vi "ContinuousCapture.vi"(8 "error in (no error)":errorcluster, 11 "Instruments in":refnum<class "Instruments.lvclass">) -> (0 "error out":errorcluster, 3 "Instruments out":refnum<class "Instruments.lvclass">)   [LabVIEW 2012, in "Instruments.lvclass"]
uses:
  Instruments.lvclass
  Instruments.lvclass/Instruments.ctl
  SpectrumCommands.ctl
  Controls/SpectrometerOphirSelector.ctl
  SpectrumWindowExit.vi
  Controls/Config.ctl
panel:
  in  "DeviceCurrent":enum16{"20mA", "50mA"}(ring)
  out "Vf":dbl format="%0.2f"
  out "Keithley":refnum<visa-resource-name>
  out "DeviceIndicator":bool
  in  "TurnOffDevice":bool
  in  "TurnOnDevice":bool
  out "Ready":bool
  in  "Int Time(ms)":i32
  in  "Enabled":bool
  in  "Exit":bool
  in  "StopCapture":bool
  in  "StartCapture":bool
  in  "Graph":cluster{"Y":dbl[], "Y":dbl[]}[](graph)
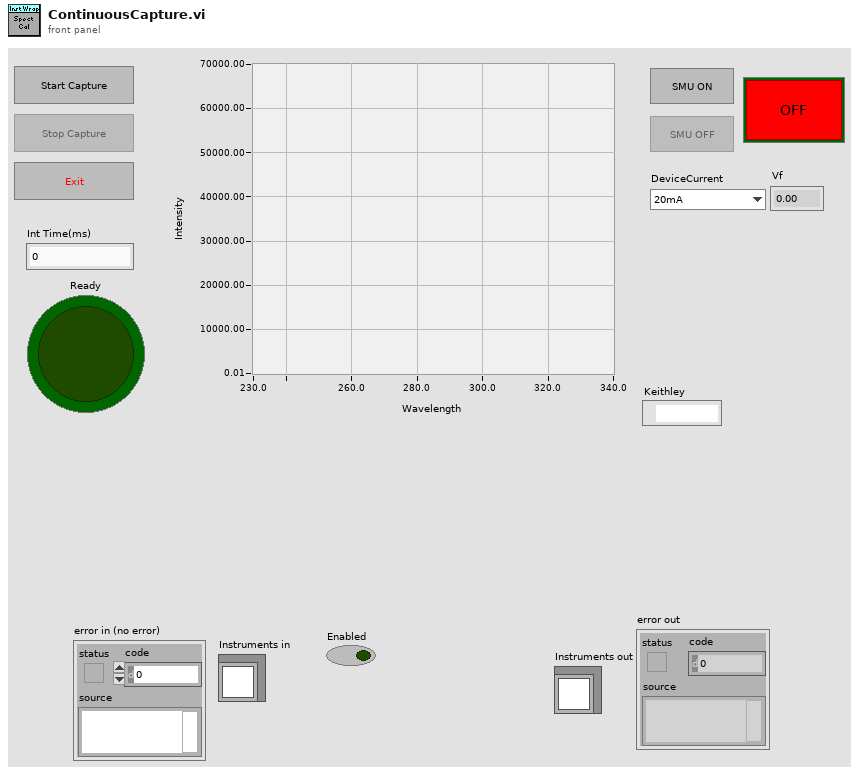
[diagram p1: front panel]
types:
  T1 = enum8{"Enabled", "Disabled", "Disabled and Grayed Out"}
  T2 = cluster{"StopCapture":refnum<vi>, "StartCapture":refnum<vi>, "Exit":refnum<vi>, "Enabled":refnum<vi>, "Ready":refnum<vi>}
  T3 = typedef "Config.ctl" = cluster{"IntTime":i32, "Samples":i32, "PowerMin":dbl, "KneeMin":dbl, "KneeMax":dbl, "Background Wl":dbl, "Settle Delay,ms":u32, "StationId":sgl}
  T4 = typedef "SpectrumCommands.ctl" = enum16{"Init", "StartCapture", "StopCapture", "Calibrate", "TurnDeviceOn", "TurnOffDevice", "Exit"}
  T5 = typedef "SpectrometerOphirSelector.ctl" = enum16{"Get Background", "Measure", "Measure50", "Raw"}
  T6 = cluster{"Wavelength":dbl[], "EL Spectrum":dbl[]}[]
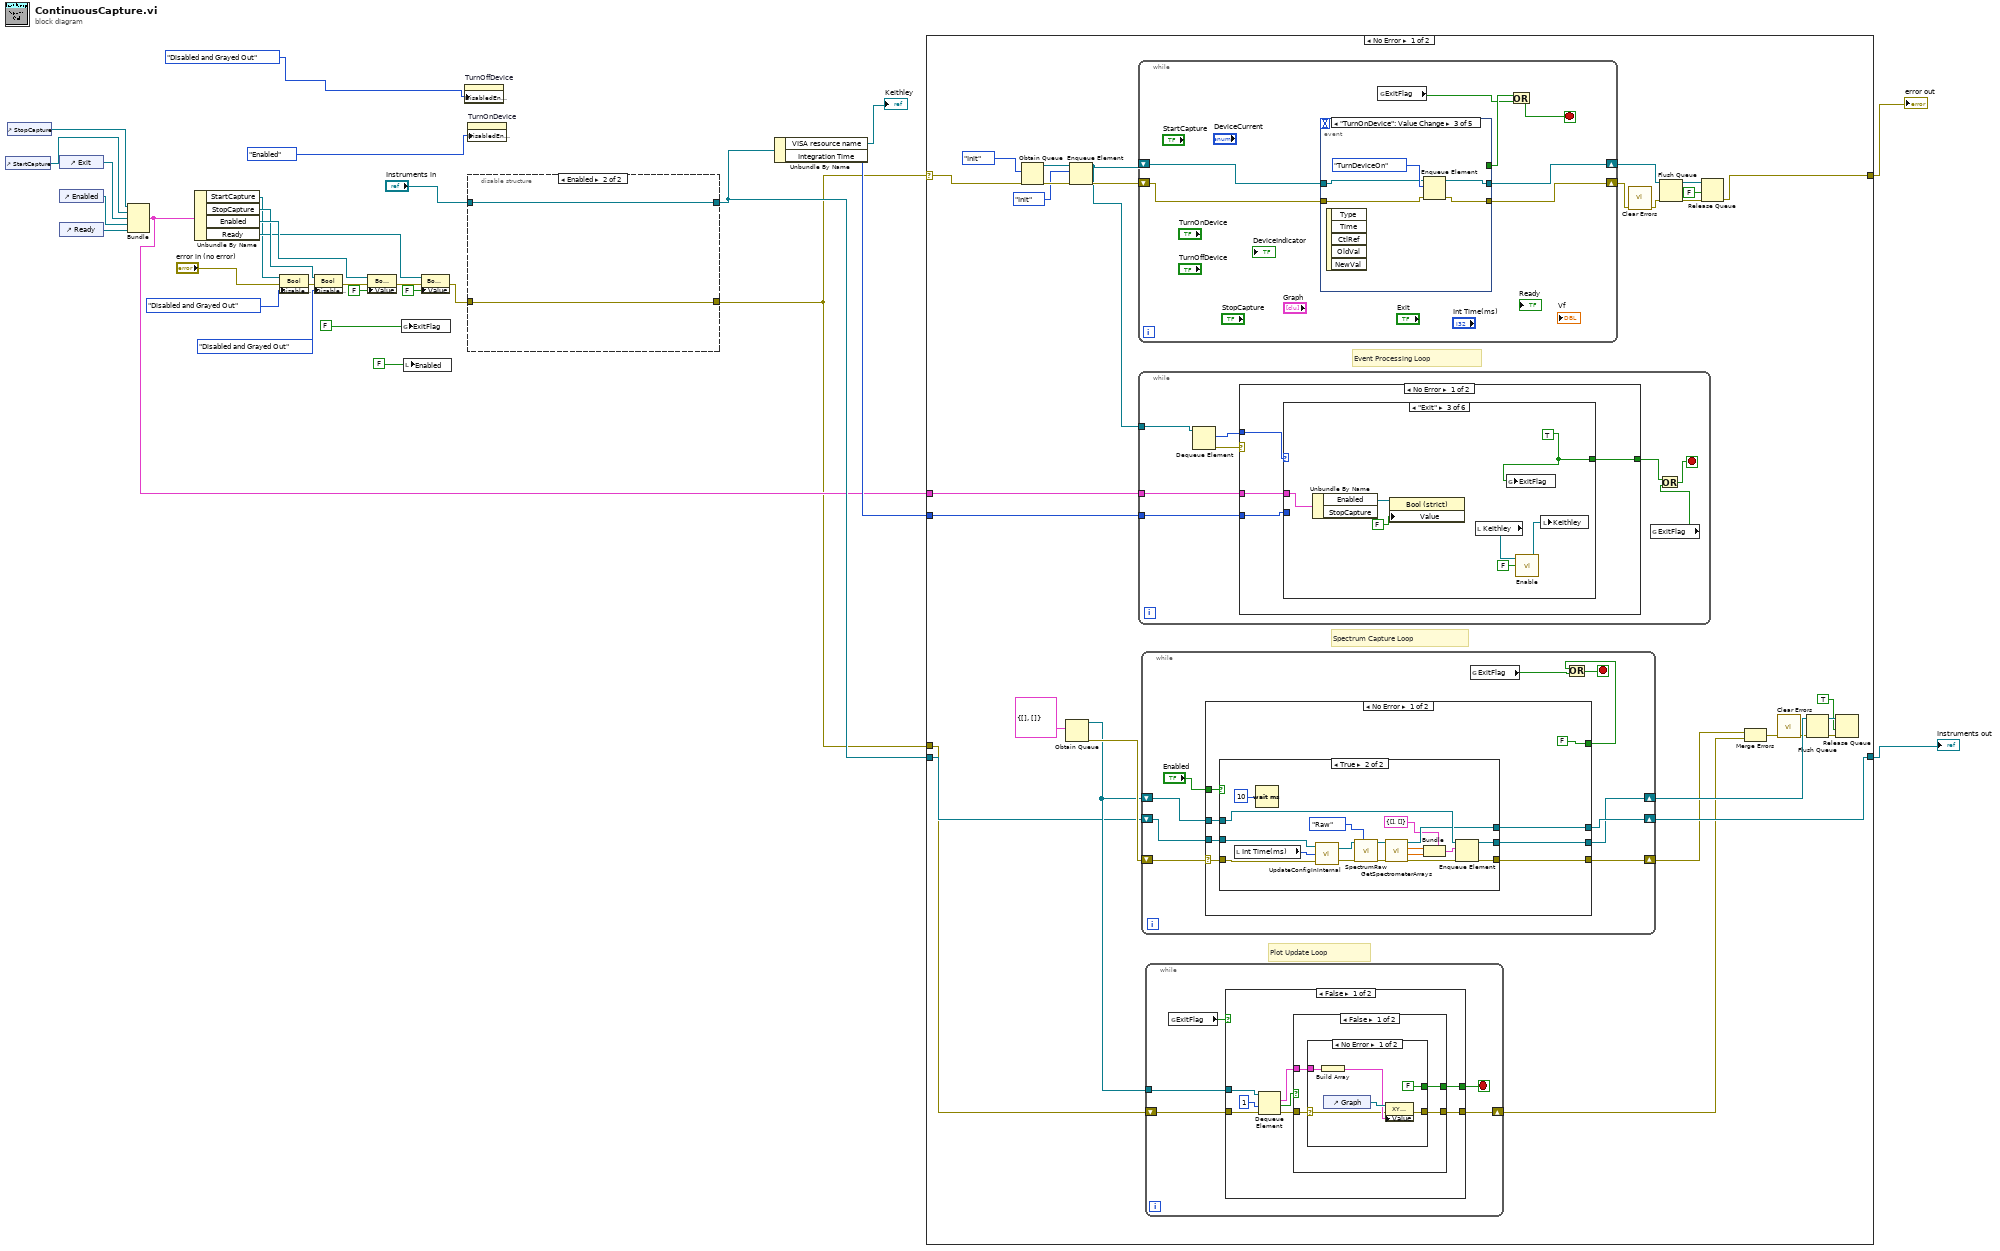
[diagram p0: block diagram]
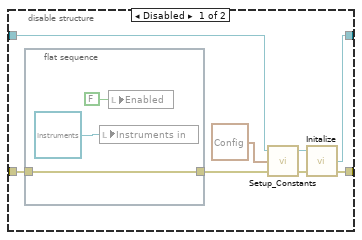
[diagram p2: hidden frame]
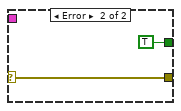
[diagram p3: hidden frame]
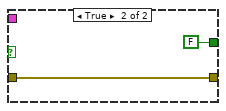
[diagram p4: hidden frame]
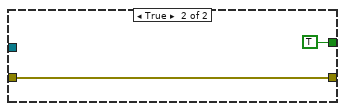
[diagram p5: hidden frame]
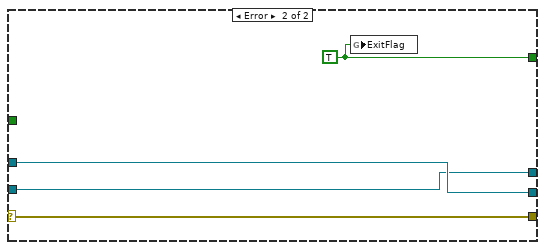
[diagram p7: hidden frame]
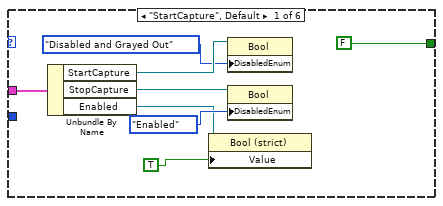
[diagram p8: hidden frame]
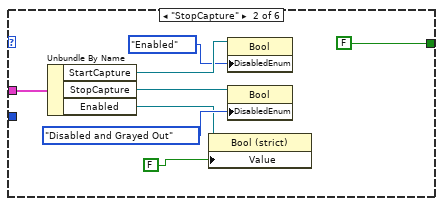
[diagram p9: hidden frame]
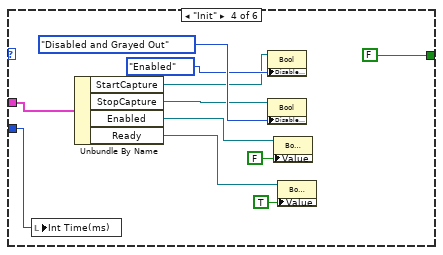
[diagram p10: hidden frame]
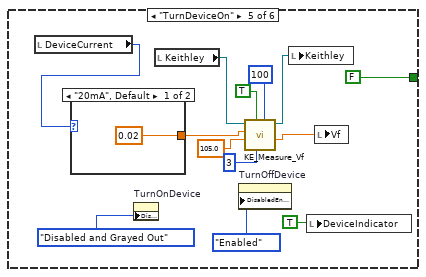
[diagram p11: hidden frame]
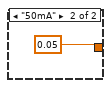
[diagram p12: hidden frame]
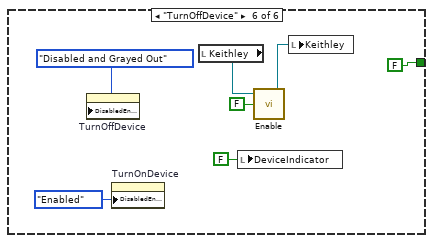
[diagram p13: hidden frame]
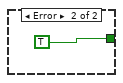
[diagram p14: hidden frame]
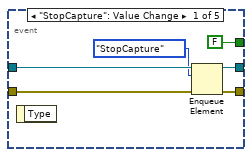
[diagram p15: hidden frame]
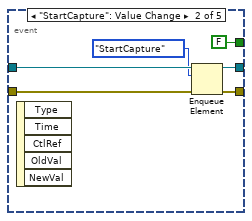
[diagram p16: hidden frame]
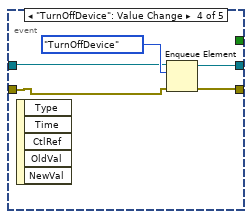
[diagram p17: hidden frame]
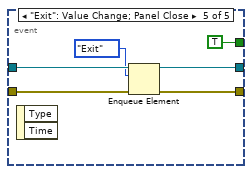
[diagram p18: hidden frame]
diagram:
  n1 = control-ref of="StartCapture"() -> (w27:refnum<vi>)
  n2 = control-ref of="StopCapture"() -> (w28:refnum<vi>)
  n3 = control-ref of="Exit"() -> (w26:refnum<vi>)
  n4 = control-ref of="Enabled"() -> (w25:refnum<vi>)
  n5 = control-ref of="Ready"() -> (w21:refnum<vi>)
  n6 = Bundle("StopCapture"=w28, "StartCapture"=w27, "Exit"=w26, "Enabled"=w25, "Ready"=w21) -> (w8:T2)  [unwired: 1 in]
  n7 = Unbundle By Name(w8) -> ("StartCapture"=w13:refnum<vi>, "StopCapture"=w17:refnum<vi>, "Enabled"=w19:refnum<vi>, "Ready"=w15:refnum<vi>)
  n8 = property class="Bool"(reference=w13, error in="error in (no error)", "DisabledEnum"=T1."Disabled and Grayed Out" ("Disabled")) -> (error out=w11:errorcluster)  [unwired: 1 out]
  n9 = property class="Bool"(reference=w17, error in=w11, "DisabledEnum"=T1."Disabled and Grayed Out" ("Disabled")) -> (error out=w10:errorcluster)  [unwired: 1 out]
  n10 = property class="Bool (strict)"(reference=w19, error in=w10, "Value"=FALSE) -> (error out=w9:errorcluster)  [unwired: 1 out]
  n11 = global write "SpectrumWindowExit.vi" "ExitFlag"(FALSE ("Enabled")) -> ()
  n12 = local write "Enabled"(FALSE ("Enabled")) -> ()
  n13 = property class="Bool (strict)"(reference=w15, error in=w9, "Value"=FALSE) -> (error out=w7:errorcluster)  [unwired: 1 out]
  n14 = property on="TurnOffDevice" class="Bool"("DisabledEnum"=T1."Disabled and Grayed Out" ("Disabled")) -> ()  [unwired: 2 in, 2 out]
  n15 = disable-structure shown="Enabled" {
    disable-tunnel: [w38 w42] -> w23
    disable-tunnel: [w37 w43] -> w6
    disable-tunnel: "Instruments in" -> [w33 w42]
    disable-tunnel: w7 -> [w31 w43]
    frame Disabled {
      n16 = flat-sequence {
        tunnel: [w40] -> w32
        tunnel: w31 -> [w40]
        frame #0 {
          n17 = local write "Instruments in"(refnum<class "Instruments.lvclass"> refnum ("Instruments in")) -> ()
          n18 = local write "Enabled"(FALSE ("Enabled")) -> ()
        }
      }
      n19 = call-dynamic "Setup_Constants.vi"("error in (no error)"=w32, "Config In"=T3 {"IntTime"=100, "Samples"=3, "PowerMin"=300.0, "KneeMin"=-20.0, "KneeMax"=20.0, "Background Wl"=275.0, "Settle Delay,ms"=0, "StationId"=0.0}, "Instruments in"=w33) -> ("error out"=w34:errorcluster, "Instruments out"=w35:refnum<class "Instruments.lvclass">)  [unwired: 1 in]
      n20 = call-dynamic "Initalize.vi"("error in (no error)"=w34, "Instruments in"=w35) -> ("error out"=w37:errorcluster, "Instruments out"=w38:refnum<class "Instruments.lvclass">)  [unwired: 2 in]
    }
    frame Enabled {
    }
  }
  n21 = property on="TurnOnDevice" class="Bool"("DisabledEnum"=T1."Enabled" ("Disabled")) -> ()  [unwired: 2 in, 2 out]
  n22 = Unbundle By Name(w23) -> ("VISA resource name"=→"Keithley":refnum<visa-resource-name>, "Integration Time"=w22:i32)
  n23 = case shown="No Error" w6 {
    selector: w6 -> [w72 w251]
    tunnel: [w62 w251] -> w30
    tunnel: [w69 w250] -> w29
    tunnel: w23 -> [w67 w250]
    tunnel: w8 -> [w44 _]
    tunnel: w6 -> [w66 _]
    tunnel: w22 -> [w46 _]
    frame No Error {
      # "Spectrum Capture Loop"
      # "Plot Update Loop"
      # "Event Processing Loop"
      n24 = Obtain Queue(element data type=SpectrumCommands."Init", error in (no error)=w72) -> (queue out=w50:refnum<queue>, error out=w49:errorcluster)  [unwired: 3 in, 1 out]
      n25 = Obtain Queue(element data type=cluster{"Wavelength":dbl[], "EL Spectrum":dbl[]} {"Wavelength"=[], "EL Spectrum"=[]}) -> (queue out=w68:refnum<queue>, error out=w70:errorcluster)  [unwired: 4 in, 1 out]
      n26 = Enqueue Element(queue=w50, element=SpectrumCommands."Init", error in (no error)=w49) -> (queue out=w45:refnum<queue>, error out=w47:errorcluster)  [unwired: 1 in, 1 out]
      n27 = while {
        shift-right: [w218] -> w63
        shift-left: w45 -> [w221]
        shift-right: [w219] -> w56
        shift-left: w47 -> [w220]
        stop <- w216 stop-if-true
        n28 = event shown="[2] \"TurnOnDevice\": Value Change" {
          selector: _ -> [_ _ _ _ _]
          dyn-events: _ -> [_ _ _ _ _]
          timeout: _ -> [_ _ _ _ _]
          tunnel: w221 -> [w227 w233 w237 w242 w249]
          tunnel: w220 -> [w226 w232 w236 w241 w248]
          tunnel: [w225 w231 w235 w240 w247] -> w219
          tunnel: [w224 w230 w234 w239 w246] -> w218
          tunnel: [FALSE ("ExitFlag") FALSE ("ExitFlag") _ _ TRUE ("ExitFlag")] -> w217
          event "StopCapture": Value Change {
            n29 = event-data() -> ()  [unwired: 1 in, 1 out]
            n30 = Enqueue Element(queue=w227, element=SpectrumCommands."StopCapture", error in (no error)=w226) -> (queue out=w224:refnum<queue>, error out=w225:errorcluster)  [unwired: 1 in, 1 out]
          }
          event "StartCapture": Value Change {
            n31 = event-data() -> ()  [unwired: 1 in, 5 out]
            n32 = Enqueue Element(queue=w233, element=SpectrumCommands."StartCapture", error in (no error)=w232) -> (queue out=w230:refnum<queue>, error out=w231:errorcluster)  [unwired: 1 in, 1 out]
          }
          event "TurnOnDevice": Value Change {
            n33 = event-data() -> ()  [unwired: 1 in, 5 out]
            n34 = Enqueue Element(queue=w237, element=SpectrumCommands."TurnDeviceOn", error in (no error)=w236) -> (queue out=w234:refnum<queue>, error out=w235:errorcluster)  [unwired: 1 in, 1 out]
          }
          event "TurnOffDevice": Value Change {
            n35 = event-data() -> ()  [unwired: 1 in, 5 out]
            n36 = Enqueue Element(queue=w242, element=SpectrumCommands."TurnOffDevice", error in (no error)=w241) -> (queue out=w239:refnum<queue>, error out=w240:errorcluster)  [unwired: 1 in, 1 out]
          }
          event "Exit": Value Change; Panel Close {
            n37 = event-data() -> ()  [unwired: 1 in, 2 out]
            n38 = Enqueue Element(queue=w249, element=SpectrumCommands."Exit", error in (no error)=w248) -> (queue out=w246:refnum<queue>, error out=w247:errorcluster)  [unwired: 1 in, 1 out]
          }
        }
        n39 = global read "SpectrumWindowExit.vi" "ExitFlag"() -> (w215:bool)
        n40 = Or(x=w217, y=w215) -> (x .or. y?=w216:bool)
      }
      n41 = while {
        tunnel: w44 -> [w151]
        tunnel: w46 -> [w147]
        tunnel: w45 -> [w146]
        stop <- w149 stop-if-true
        n42 = Dequeue Element(queue=w146) -> (element=w152:T4, error out=w153:errorcluster)  [unwired: 2 in, 2 out]
        n43 = case shown="No Error" w153 {
          tunnel: w152 -> [w157 _]
          tunnel: w151 -> [w156 _]
          tunnel: [w155 TRUE ("x")] -> w150
          tunnel: w147 -> [w154 _]
          frame No Error {
            n44 = case shown="\"Exit\"" w157 {
              tunnel: w156 -> [w165 w168 w180 w184 _ _]
              tunnel: [FALSE ("x") FALSE ("x") w177 FALSE ("x") FALSE ("x") FALSE ("x")] -> w155
              tunnel: w154 -> [_ _ _ w190 _ _]
              frame "StartCapture", Default {
                n45 = Unbundle By Name(w165) -> ("StartCapture"=w164:refnum<vi>, "StopCapture"=w162:refnum<vi>, "Enabled"=w160:refnum<vi>)
                n46 = property class="Bool (strict)"(reference=w160, "Value"=TRUE) -> ()  [unwired: 1 in, 2 out]
                n47 = property class="Bool"(reference=w164, "DisabledEnum"=T1."Disabled and Grayed Out" ("Disabled")) -> ()  [unwired: 1 in, 2 out]
                n48 = property class="Bool"(reference=w162, "DisabledEnum"=T1."Enabled" ("Disabled")) -> ()  [unwired: 1 in, 2 out]
              }
              frame "StopCapture" {
                n49 = Unbundle By Name(w168) -> ("StartCapture"=w173:refnum<vi>, "StopCapture"=w171:refnum<vi>, "Enabled"=w169:refnum<vi>)
                n50 = property class="Bool (strict)"(reference=w169, "Value"=FALSE) -> ()  [unwired: 1 in, 2 out]
                n51 = property class="Bool"(reference=w173, "DisabledEnum"=T1."Enabled" ("Disabled")) -> ()  [unwired: 1 in, 2 out]
                n52 = property class="Bool"(reference=w171, "DisabledEnum"=T1."Disabled and Grayed Out" ("Disabled")) -> ()  [unwired: 1 in, 2 out]
              }
              frame "Exit" {
                w177 = TRUE ("x")
                n53 = Unbundle By Name(w180) -> ("Enabled"=w179:refnum<vi>)  [unwired: 1 out]
                n54 = property class="Bool (strict)"(reference=w179, "Value"=FALSE) -> ()  [unwired: 1 in, 2 out]
                n55 = local read "Keithley"() -> (w176:refnum<visa-resource-name>)
                n56 = global write "SpectrumWindowExit.vi" "ExitFlag"(w177) -> ()
                n57 = call "Enable.vi"("Enable Output (T: Enable)"=FALSE, "VISA resource name"=w176) -> ("VISA resource name out"=w175:refnum<visa-resource-name>)  [unwired: 1 in, 1 out]
                n58 = local write "Keithley"(w175) -> ()
              }
              frame "Init" {
                n59 = local write "Int Time(ms)"(w190) -> ()
                n60 = Unbundle By Name(w184) -> ("StartCapture"=w181:refnum<vi>, "StopCapture"=w186:refnum<vi>, "Enabled"=w188:refnum<vi>, "Ready"=w183:refnum<vi>)
                n61 = property class="Bool"(reference=w181, "DisabledEnum"=T1."Enabled" ("Disabled")) -> ()  [unwired: 1 in, 2 out]
                n62 = property class="Bool"(reference=w186, "DisabledEnum"=T1."Disabled and Grayed Out" ("Disabled")) -> ()  [unwired: 1 in, 2 out]
                n63 = property class="Bool (strict)"(reference=w188, "Value"=FALSE) -> ()  [unwired: 1 in, 2 out]
                n64 = property class="Bool (strict)"(reference=w183, "Value"=TRUE) -> ()  [unwired: 1 in, 2 out]
              }
              frame "TurnDeviceOn" {
                n65 = local read "DeviceCurrent"() -> (w204:enum16{"20mA", "50mA"})
                n66 = case shown="\"20mA\", Default" w204 {
                  tunnel: [0.02 0.05] -> w203
                  frame "20mA", Default {
                  }
                  frame "50mA" {
                  }
                }
                n67 = property on="TurnOnDevice" class="Bool"("DisabledEnum"=T1."Disabled and Grayed Out" ("Disabled")) -> ()  [unwired: 2 in, 2 out]
                n68 = local read "Keithley"() -> (w201:refnum<visa-resource-name>)
                n69 = property on="TurnOffDevice" class="Bool"("DisabledEnum"=T1."Enabled" ("Disabled")) -> ()  [unwired: 2 in, 2 out]
                n70 = call "KE_Measure_Vf.vi"("Settle Delay"=u32 100, "Samples"=3, "Keep On"=TRUE, "Compliance"=105.0, "Current(A)"=w203, "KE_In"=w201) -> ("Vf"=w196:dbl, "KE_Out"=w197:refnum<visa-resource-name>)  [unwired: 3 in, 1 out]
                n71 = local write "Keithley"(w197) -> ()
                n72 = local write "DeviceIndicator"(TRUE ("DeviceIndicator")) -> ()
                n73 = local write "Vf"(w196) -> ()
              }
              frame "TurnOffDevice" {
                n74 = property on="TurnOffDevice" class="Bool"("DisabledEnum"=T1."Disabled and Grayed Out" ("Disabled")) -> ()  [unwired: 2 in, 2 out]
                n75 = property on="TurnOnDevice" class="Bool"("DisabledEnum"=T1."Enabled" ("Disabled")) -> ()  [unwired: 2 in, 2 out]
                n76 = local read "Keithley"() -> (w213:refnum<visa-resource-name>)
                n77 = local write "DeviceIndicator"(FALSE ("DeviceIndicator")) -> ()
                n78 = call "Enable.vi"("Enable Output (T: Enable)"=FALSE, "VISA resource name"=w213) -> ("VISA resource name out"=w212:refnum<visa-resource-name>)  [unwired: 1 in, 1 out]
                n79 = local write "Keithley"(w212) -> ()
              }
            }
          }
          frame Error {
          }
        }
        n80 = global read "SpectrumWindowExit.vi" "ExitFlag"() -> (w148:bool)
        n81 = Or(x=w150, y=w148) -> (x .or. y?=w149:bool)
      }
      n82 = while {
        shift-right: [w108] -> w57
        shift-left: w68 -> [w109]
        shift-right: [w110] -> w69
        shift-left: w67 -> [w111]
        shift-right: [w107] -> w54
        shift-left: w70 -> [w106]
        stop <- w105 stop-if-true
        n83 = case shown="No Error" w106 {
          selector: w106 -> [w114 w143]
          tunnel: "Enabled" -> [w120 _]
          tunnel: w111 -> [w119 w144]
          tunnel: [w118 w144] -> w110
          tunnel: w109 -> [w117 w145]
          tunnel: [w116 w145] -> w108
          tunnel: [w115 w143] -> w107
          tunnel: [FALSE ("ExitFlag") w142] -> w104
          frame No Error {
            n84 = case shown="True" w120 {
              tunnel: w119 -> [w122 w131]
              tunnel: [w122 w138] -> w118
              tunnel: w117 -> [w123 w141]
              tunnel: [w123 w139] -> w116
              tunnel: [w121 w136] -> w115
              tunnel: w114 -> [w121 w129]
              frame False {
              }
              frame True {
                n85 = local read "Int Time(ms)"() -> (w130:i32)
                n86 = Wait (ms)(milliseconds to wait=u32 10) -> ()  [unwired: 1 out]
                n87 = call-dynamic "UpdateConfigInInternal.vi"("error in (no error)"=w129, "IntTime"=w130, "Instruments in"=w131) -> ("error out"=w127:errorcluster, "Instruments out"=w128:refnum<class "Instruments.lvclass">)
                n88 = call-dynamic "SpectrumRaw.vi"("Type"=SpectrometerOphirSelector."Raw", "error in (no error)"=w127, "Instruments in"=w128) -> ("error out"=w126:errorcluster, "Instruments out"=w125:refnum<class "Instruments.lvclass">)  [unwired: 4 in, 3 out]
                n89 = call-dynamic "GetSpectrometerArrays.vi"("error in (no error)"=w126, "Instruments in"=w125) -> ("error out"=w137:errorcluster, "Spectrum"=w132:dbl[], "Wavelength"=w133:dbl[], "Instruments out"=w138:refnum<class "Instruments.lvclass">)  [unwired: 6 in]
                n90 = Bundle(cluster=cluster{"Wavelength":dbl[], "EL Spectrum":dbl[]} {"Wavelength"=[], "EL Spectrum"=[]}, "Wavelength"=w133, "EL Spectrum"=w132) -> (w140:cluster{"Wavelength":dbl[], "EL Spectrum":dbl[]})
                n91 = Enqueue Element(queue=w141, element=w140, error in (no error)=w137) -> (queue out=w139:refnum<queue>, error out=w136:errorcluster)  [unwired: 1 in, 1 out]
              }
            }
          }
          frame Error {
            w142 = TRUE ("ExitFlag")
            n92 = global write "SpectrumWindowExit.vi" "ExitFlag"(w142) -> ()
          }
        }
        n93 = global read "SpectrumWindowExit.vi" "ExitFlag"() -> (w103:bool)
        n94 = Or(x=w104, y=w103) -> (x .or. y?=w105:bool)
      }
      n95 = while {
        tunnel: w68 -> [w74]
        shift-right: [w78] -> w53
        shift-left: w66 -> [w76]
        stop <- w75 stop-if-true
        n96 = global read "SpectrumWindowExit.vi" "ExitFlag"() -> (w77:bool)
        n97 = case shown="False" w77 {
          tunnel: [w84 w102] -> w78
          tunnel: w76 -> [w81 w102]
          tunnel: [w83 TRUE] -> w75
          tunnel: w74 -> [w82 _]
          frame False {
            n98 = Dequeue Element(queue=w82, timeout in ms (-1)=1, error in (no error)=w81) -> (element=w85:cluster{"Wavelength":dbl[], "EL Spectrum":dbl[]}, timed out?=w79:bool, error out=w86:errorcluster)  [unwired: 1 out]
            n99 = case shown="False" w79 {
              tunnel: w86 -> [w90 w100]
              tunnel: w85 -> [w89 _]
              tunnel: [w88 w100] -> w84
              tunnel: [w87 FALSE] -> w83
              frame False {
                n100 = case shown="No Error" w90 {
                  selector: w90 -> [w92 w97]
                  tunnel: w89 -> [w96 _]
                  tunnel: [FALSE TRUE] -> w87
                  tunnel: [w91 w97] -> w88
                  frame No Error {
                    n101 = Build Array(w96) -> (w93:T6)
                    n102 = control-ref of="Graph"() -> (w94:refnum<vi>)
                    n103 = property class="XYGraph (strict)"(reference=w94, error in=w92, "Value"=w93) -> (error out=w91:errorcluster)  [unwired: 1 out]
                  }
                  frame Error {
                  }
                }
              }
              frame True {
              }
            }
          }
          frame True {
          }
        }
      }
      n104 = call <vilib>:"Clear Errors.vi"("error in (no error)"=w56) -> ("error out"=w55:errorcluster)  [unwired: 6 in]
      n105 = Flush Queue(queue=w63, error in (no error)=w55) -> (queue out=w65:refnum<queue>, error out=w64:errorcluster)  [unwired: 1 out]
      n106 = Release Queue(queue=w65, force destroy? (F)=FALSE, error in (no error)=w64) -> (error out=w62:errorcluster)  [unwired: 2 out]
      n107 = Merge Errors(w54, w53) -> (w52:errorcluster)
      n108 = call <vilib>:"Clear Errors.vi"("error in (no error)"=w52) -> ("error out"=w51:errorcluster)  [unwired: 6 in]
      n109 = Flush Queue(queue=w57, error in (no error)=w51) -> (queue out=w60:refnum<queue>, error out=w59:errorcluster)  [unwired: 1 out]
      n110 = Release Queue(queue=w60, force destroy? (F)=TRUE, error in (no error)=w59) -> ()  [unwired: 3 out]
    }
    frame Error {
    }
  }
  "error out" <- w30
  "Instruments out" <- w29
